vi "Create AES Cipher.vi"(8 "error in (no error)":errorcluster, 10 "Operation Mode":T1=enum."CBC", 11 "Cipher Key":string) -> (0 "error out":errorcluster, 3 "AES out":refnum<class "AES.lvclass">)   [LabVIEW 2020, in "AES.lvclass"]
uses:
  AES.lvclass
  Ton Plomp Encryption/AES-Modes.ctl
  AES.lvclass/AES.ctl
  Ton Plomp Encryption/Encryption.lvlib
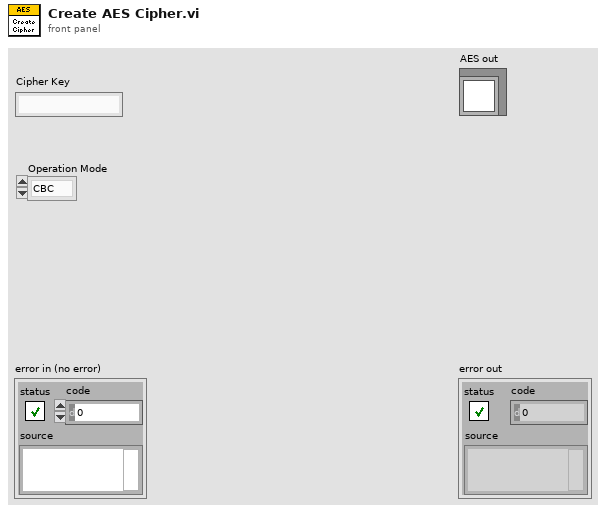
[diagram p1: front panel]
types:
  T1 = typedef "Encryption.lvlib/AES-Modes.ctl" = enum16{"ECB", "CBC", "CFB128", "OFB"}
  T2 = cluster{bool, i32, "String to Prepend to source (\"\")":string}
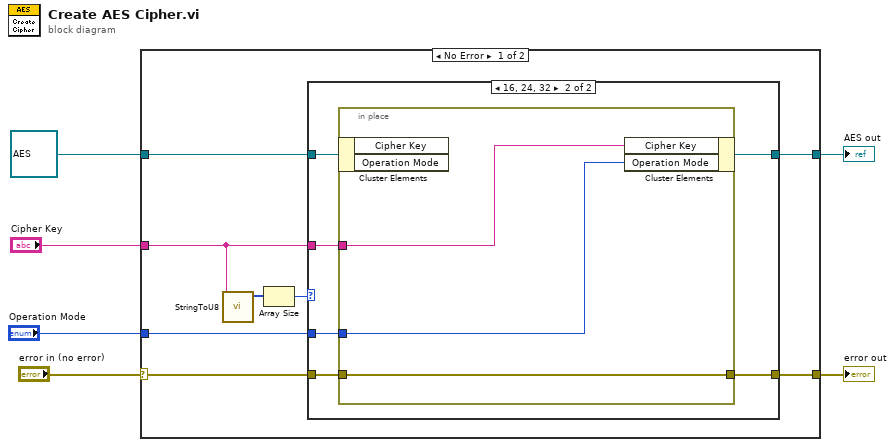
[diagram p0: block diagram]
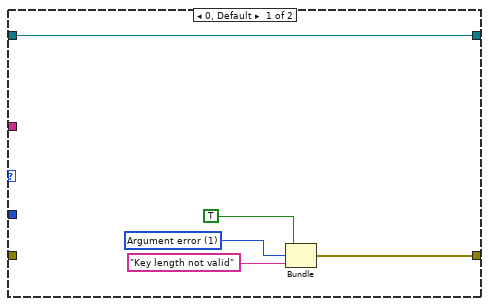
[diagram p2: hidden frame]
diagram:
  n1 = case shown="No Error" "error in (no error)" {
    selector: "error in (no error)" -> [w7 w30]
    tunnel: [w8 w30] -> w5
    tunnel: [w11 w29] -> w3
    tunnel: refnum<class "AES.lvclass"> refnum ("AES in") -> [w12 w29]
    tunnel: "Operation Mode" -> [w10 _]
    tunnel: "Cipher Key" -> [w9 _]
    frame No Error {
      n2 = call "StringToU8.vi"("HEX text in"=w9) -> ("ArrayU8 out"=w13:u8[])  [unwired: 9 in, 1 out]
      n3 = Array Size(array=w13) -> (size(s)=w14:i32)
      n4 = case shown="16, 24, 32" w14 {
        tunnel: w12 -> [w16 w25]
        tunnel: [w16 w24] -> w11
        tunnel: w10 -> [_ w23]
        tunnel: w9 -> [_ w22]
        tunnel: [w15 w20] -> w8
        tunnel: w7 -> [_ w21]
        frame 0, Default {
          w18 = 1 items=["No error", "Argument error", "Memory is full", "Out of zone", "End of file", "File already open", "Generic file I/O error", "File not found", "File permission error", "Disk is full", "Duplicate path", "Too many files open", "System feature not enabled", "Resource file not found", "Cannot add resource", "Resource not found", "Image not found", "Image memory error", "Pen does not exist", "Config type invalid", "Config token not found", "Config parse error", "Config memory error", "Bad external code format", "Bad external code offset", "External code not present", "Null window", "Destroy window error", "Null menu", "Print aborted", "Bad print record", "Print driver error", "Windows error during printing", "Memory error during printing", "Print dialog error", "Generic print error", "Invalid device refnum", "Device not found", "Device parameter error", "Device unit error", "Cannot open device", "Device call aborted", "Generic error", "Cancelled by user", "Object ID too low", "Object ID too high", "Object not in heap", "Unknown heap", "Unknown object (invalid DefProc)", "Unknown object (DefProc not in table)", "Message out of range", "Invalid (null) method", "Unknown message", "Manager call not supported", "Bad address", "Network operation in progress", "Network operation timed out", "Connection is busy", "Network attribute not supported", "Network error", "Address in use", "System out of memory", "Connection aborted", "Connection refused", "Not connected", "Already connected", "Connection closed", "Initialization error (interapplication manager)", "Bad occurrence", "Wait on unbound occurrence handler", "Occurrence queue overflow", "Datalog type conflict", "Unused", "Unrecognized type (interapplication manager)", "Memory corrupt", "Failed to make temporary DLL", "Old CIN version", "Drag socket not found", "Failed to load drop-object", "Failed to register OLE object", "Failed to release OLE object", "Format specifier type mismatch", "Unknown format specifier", "Too few format specifiers", "Too many format specifiers", "Scan failed", "Newer CIN version", "Error converting to variant", "Runtime menu error", "Password tampered", "Variant attribute not found", "Incompatible variant data type", "Event data is not available", "Event Store is not present", "Occurrence is not found", "Event Queue is not created", "Event info is not available", "Refnum passed is NULL", "Error retrieving Class GUID", "Error retrieving CoClass GUID", "Error retrieving TypeLib GUID.", "Bad built application magic bytes.", "Specific driver is different from the specific driver associated with the Logical Name.", "There is no session opened to the class driver.", "Max Error", "MAX - Error with config objects", "MAX - Error loading configuration", "MAX - Group not supported"]
          n5 = Bundle(TRUE, w18, "String to Prepend to source (\"\")"="Key length not valid" ("String to Prepend to source (\"\")")) -> (w15:T2)  [unwired: 1 in]
        }
        frame 16, 24, 32 {
          n6 = in-place {
            in-place-border: w23 -> [w28]
            in-place-border: w22 -> [w26]
            in-place-border: w21 -> [w27]
            in-place-border: [w27] -> w20
            n7 = in-place-cluster #1(w25) -> ()  [unwired: 2 out]
            n8 = in-place-cluster #1("Cipher Key"=w26, "Operation Mode"=w28) -> (w24:refnum<class "AES.lvclass">)
          }
        }
      }
    }
    frame Error {
    }
  }
  "error out" <- w5
  "AES out" <- w3
